vi "Get Base Name.vi"(3 "Unique Name":string) -> (1 "Base Name":string)   [LabVIEW 2019, in "Tree.lvclass"]
uses:
  Tree.lvclass
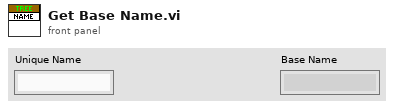
[diagram p1: front panel]
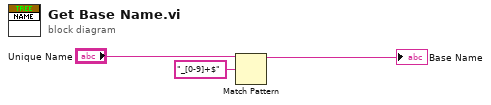
[diagram p0: block diagram]
diagram:
  n1 = Match Pattern(string="Unique Name", regular expression="_[0-9]+$") -> (before substring=→"Base Name":string)  [unwired: 1 in, 3 out]
